vi "{{Msg}}.vi"(6 "Error":errorcluster, 7 "Actor Msg":refnum<class "Actor Msg.lvclass">, 9 "Payload":T1, 10 "Msg Attribs":T2 {"Listen Absolute Time" format="%<%x %.3X>T"; "Tell Absolute Time" format="%<%x %.3X>T"}, 11 "Actor":T5) -> (1 "Payload":T1, 2 "Msg Attribs":T2 {"Listen Absolute Time" format="%<%x %.3X>T"; "Tell Absolute Time" format="%<%x %.3X>T"}, 3 "Actor":T5, 4 "Error":errorcluster, 5 "Actor Msg":refnum<class "Actor Msg.lvclass">)   [LabVIEW 2020, in "_Template.lvlib" / "{{Msg}}.lvlib" / "Actor Msg.lvclass"]
uses:
  Actor Msg.lvclass
  jettl/jettl/Msg/Msg.lvclass
  jettl/jettl/Actor Layer/Actor Layer.lvclass
  jettl/jettl/Msg.ctl
  jettl/jettl/jettl.lvlib
  jettl/jettl/Post Setup.ctl
  jettl/jettl/Pre Setup.ctl
  jettl/jettl/Msg Set.ctl
  jettl/jettl/Lifecycle.ctl
  jettl/jettl/Actor Attribs.ctl
  jettl/jettl/Children.ctl
  jettl/jettl/Actor.ctl
  jettl/jettl/Msg Attribs.ctl
  jettl/jettl/Origin.ctl
  jettl/jettl/Layer Type.ctl
  jettl/jettl/Layer Attribs.ctl
  jettl/jettl/Layer Map.ctl
  jettl/jettl/Implemented Map.ctl
  Payload.ctl
  {{Msg}}.lvlib
panel:
  # "This front panel should not be manipulated."
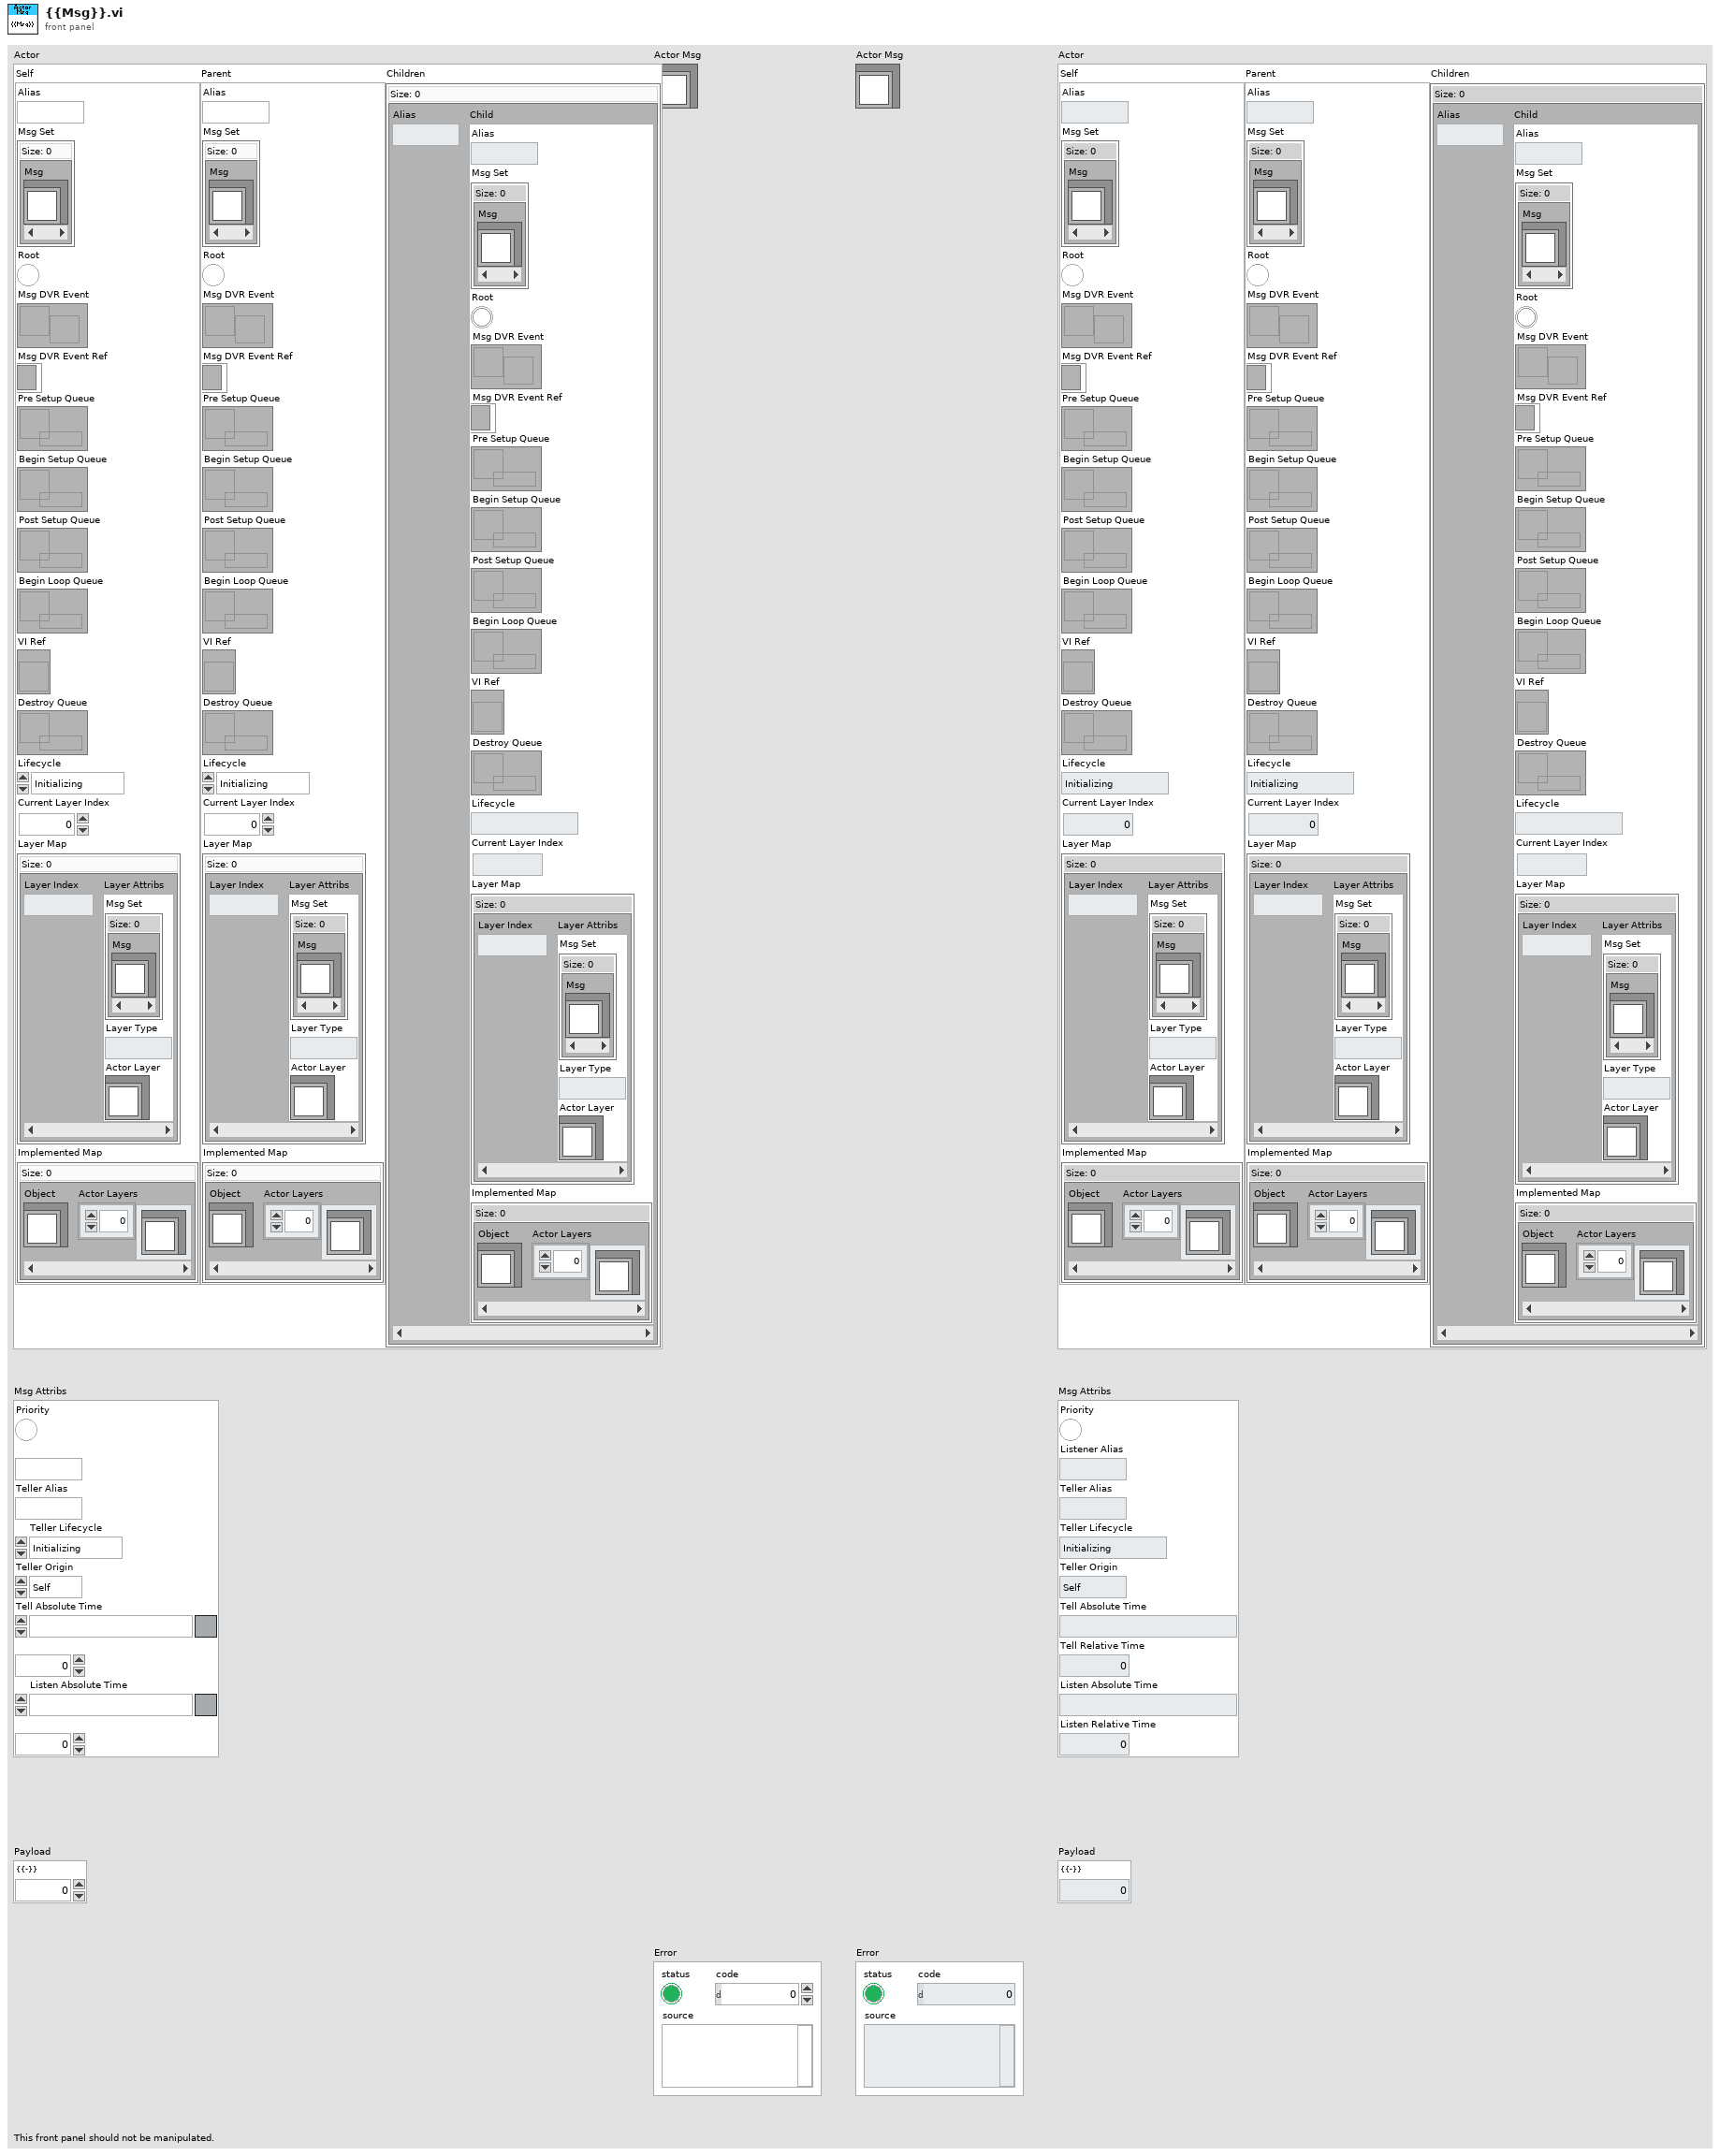
[diagram p1: front panel]
types:
  T1 = typedef "_Template.lvlib/{{Msg}}.lvlib/Payload.ctl" = cluster{"{{-}}":u8}
  T2 = typedef "jettl.lvlib/Msg Attribs.ctl" = cluster{"Priority":bool, "Listener Alias":string, "Teller Alias":string, "Teller Lifecycle":T3, "Teller Origin":T4, "Tell Absolute Time":timestamp, "Tell Relative Time":dbl, "Listen Absolute Time":timestamp, "Listen Relative Time":dbl}
  T3 = typedef "jettl.lvlib/Lifecycle.ctl" = enum16{"Initializing", "Setting Up", "Starting", "Running", "Stopping", "Tearing Down", "Terminated"}
  T4 = typedef "jettl.lvlib/Origin.ctl" = enum16{"Self", "Parent", "Child"}
  T5 = typedef "jettl.lvlib/Actor.ctl" = cluster{"Self":T6, "Parent":T6, "Children":T12}
  T6 = typedef "jettl.lvlib/Actor Attribs.ctl" = cluster{"Alias":string, "Msg Set":T7, "Root":bool, "Msg DVR Event":refnum<user-event>, "Msg DVR Event Ref":refnum<event-registration>, "Pre Setup Queue":refnum<queue>, "Begin Setup Queue":refnum<queue>, "Post Setup Queue":refnum<queue>, "Begin Loop Queue":refnum<queue>, "VI Ref":refnum<vi>, "Destroy Queue":refnum<queue>, "Lifecycle":T3, "Current Layer Index":i32, "Layer Map":T8, "Implemented Map":T11}
  T7 = typedef "jettl.lvlib/Msg Set.ctl" = set{refnum<class "Msg.lvclass">}
  T8 = typedef "jettl.lvlib/Layer Map.ctl" = map{i32, T9}
  T9 = typedef "jettl.lvlib/Layer Attribs.ctl" = cluster{"Msg Set":T7, "Layer Type":T10, "Actor Layer":refnum<class "Actor Layer.lvclass">}
  T10 = typedef "jettl.lvlib/Layer Type.ctl" = enum16{"Base", "InnerGlobal", "InnerLocal", "Outer"}
  T11 = typedef "jettl.lvlib/Implemented Map.ctl" = map{refnum<class>, refnum<class "Actor Layer.lvclass">[]}
  T12 = typedef "jettl.lvlib/Children.ctl" = map{string, T6}
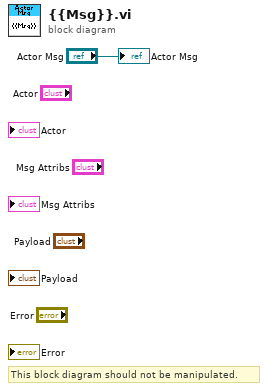
[diagram p0: block diagram]
diagram:
  # "This block diagram should not be manipulated."
  "Actor Msg" <- "Actor Msg"
